vi "WaitingTestSeq.vi"(0 "TestSeqClass in":refnum<class "TestSeqClass.lvclass">, 11 "error in (no error)":errorcluster) -> (4 "TestSeqClass out":refnum<class "TestSeqClass.lvclass">, 8 "Valid":bool, 15 "error out":errorcluster)   [LabVIEW 2019]
uses:
  TestSeqClass.lvclass
  Typedef/TestTypeSelect.ctl
  TestSeqClass.lvclass/TestSeqClass.ctl
  TestMeasureStep/TestMeasureStep.lvclass
panel:
  in  "TestType":T1
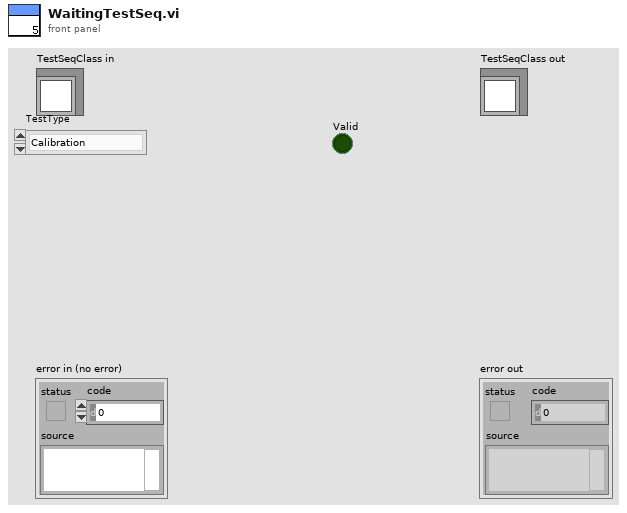
[diagram p1: front panel]
types:
  T1 = typedef "TestTypeSelect.ctl" = enum16{"Calibration", "Testing"}
  T2 = typedef "TestSeqType.ctl" = refnum<class "TestMeasureStep.lvclass">[]
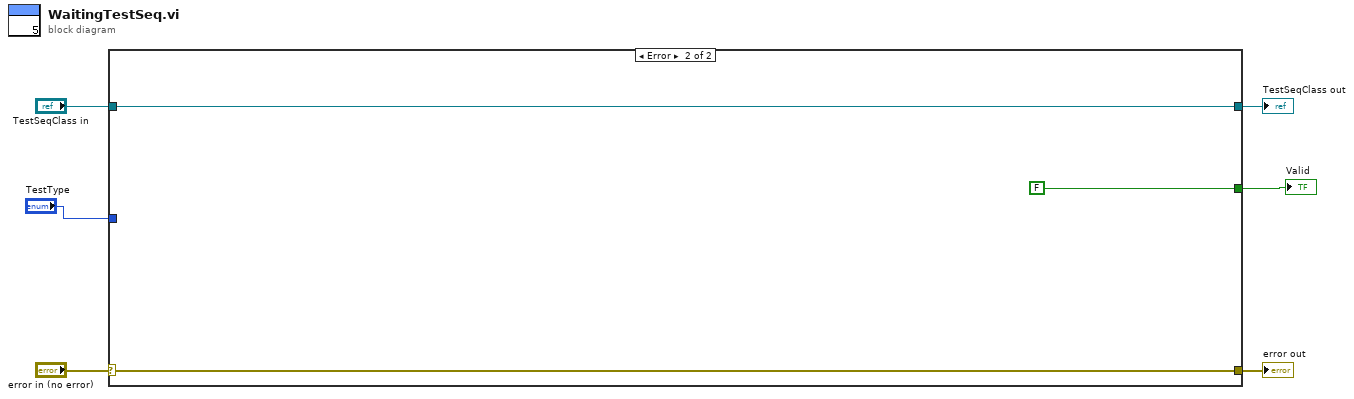
[diagram p0: block diagram]
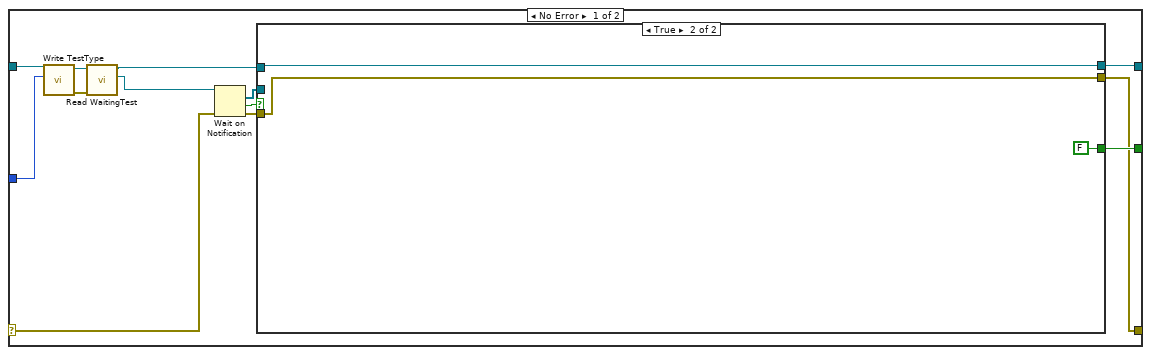
[diagram p2: hidden frame]
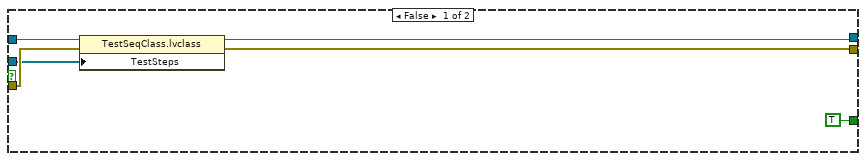
[diagram p3: hidden frame]
diagram:
  n1 = case shown="Error" "error in (no error)" {
    selector: "error in (no error)" -> [w16 w31]
    tunnel: [w17 w31] -> w5
    tunnel: [w18 w30] -> w3
    tunnel: "TestSeqClass in" -> [w12 w30]
    tunnel: [w19 FALSE] -> w2
    tunnel: "TestType" -> [w13 _]
    frame No Error {
      n2 = call-dynamic "Write TestType.vi"("TestType"=w13, "TestSeqClass in"=w12) -> ("error out"=w10:errorcluster, "TestSeqClass out"=w11:refnum<class "TestSeqClass.lvclass">)  [unwired: 8 in]
      n3 = call "Read WaitingTest.vi"("error in (no error)"=w10, "TestSeqClass in"=w11) -> ("WaitingTestSeq"=w8:refnum<notifier>, "TestSeqClass out"=w9:refnum<class "TestSeqClass.lvclass">)  [unwired: 7 in, 1 out]
      n4 = Wait on Notification(notifier=w8, error in (no error)=w16) -> (notification=w7:T2, timed out?=w14:bool, error out=w15:errorcluster)  [unwired: 2 in, 1 out]
      n5 = case shown="True" w14 {
        tunnel: [TRUE FALSE] -> w19
        tunnel: [w22 w27] -> w18
        tunnel: [w21 w28] -> w17
        tunnel: w9 -> [w25 w27]
        tunnel: w15 -> [w24 w28]
        tunnel: w7 -> [w23 _]
        frame False {
          n6 = property class="TestSeqClass.lvclass"(reference=w25, error in=w24, "TestSteps"=w23) -> (reference out=w22:refnum<class "TestSeqClass.lvclass">, error out=w21:errorcluster)
        }
        frame True {
        }
      }
    }
    frame Error {
    }
  }
  "error out" <- w5
  "TestSeqClass out" <- w3
  "Valid" <- w2
